vi "valve_controll.vi"() -> ()   [LabVIEW 2011]
uses:
  <vilib>/LabVIEW Interface for Arduino/Type Defs/Pin Mode.ctl
  <vilib>/LabVIEW Interface for Arduino/LabVIEW Interface for Arduino.lvlib
panel:
  in  "Cooling Down Time (min)":dbl=20.0 caption="Time Target (s)"
  out "Elapsed Time (s)":dbl
  out "x > y?":bool
  in  "Back Valve Time (min)":dbl=20.0 caption="Time Target (s)"
  in  "Chromatogram Time (min)":dbl=20.0 caption="Time Target (s)"
  in  "VISA resource":refnum<visa-resource-name>
  in  "Digital I/O Pin":u8
  in  "Value (0)":u8
  in  "Stop":bool
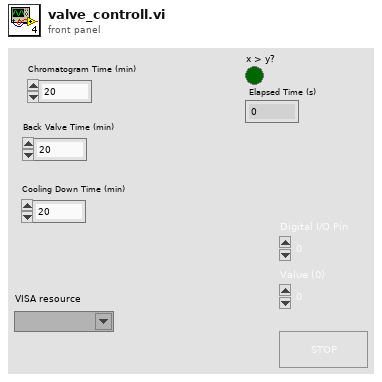
[diagram p1: front panel]
types:
  T1 = typedef "LabVIEW Interface for Arduino.lvlib/Pin Mode.ctl" = enum8{"Input", "Output"}
  T2 = typedef "LabVIEW Interface for Arduino.lvlib/Arduino Resource.ctl" = cluster{"VISA resource":refnum<visa-resource-name>, "Board Type":T3, "Connection Type":enum8{"USB / Serial"}, "Bytes Per Packet (15)":u8}
  T3 = typedef "LabVIEW Interface for Arduino.lvlib/Board Type.ctl" = enum16{"Uno", "Dimuelanove w/Atmega 328", "Mega 2560"}
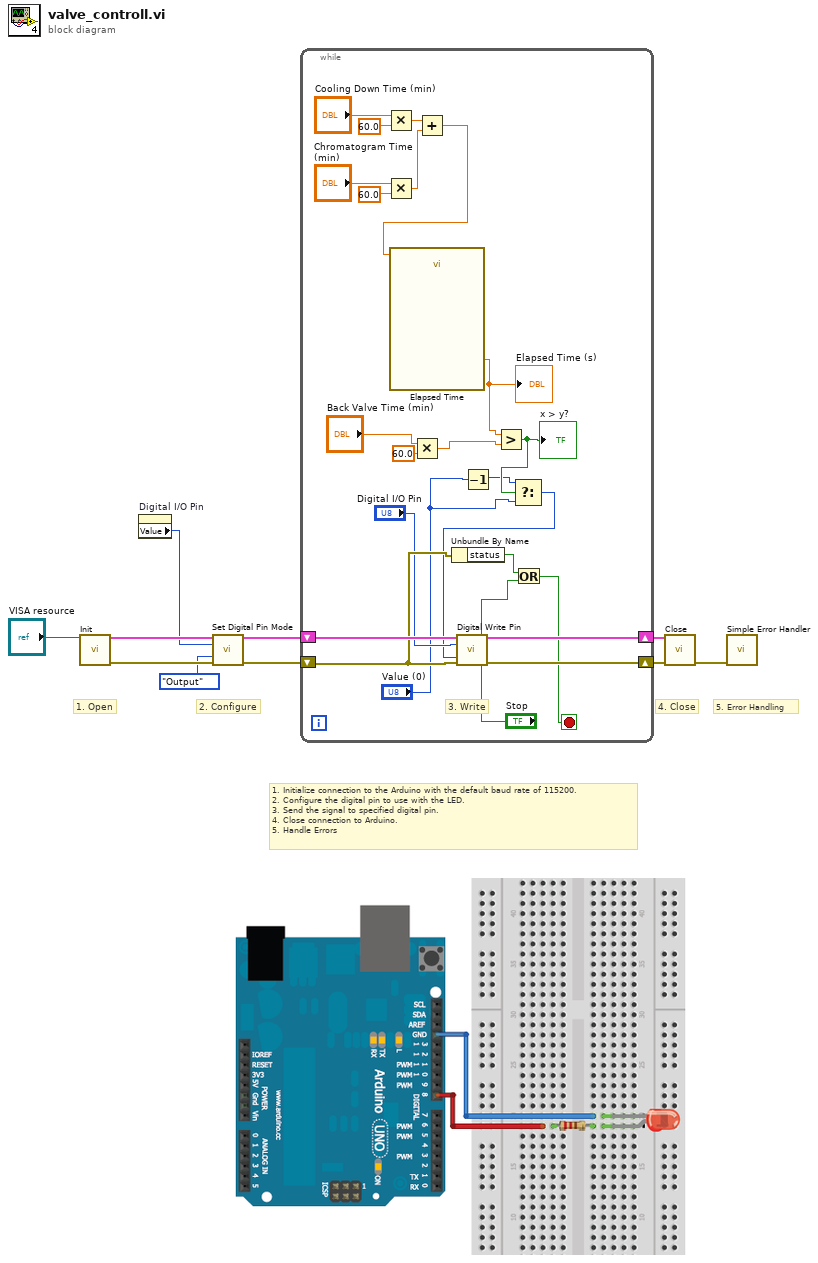
[diagram p0: block diagram]
diagram:
  # "5. Error Handling"
  # "4. Close"
  # "2. Configure"
  # "1. Open"
  # "1. Initialize connection to the Arduino with the default baud rate of 115200.\n2. Configure the digital pin to use with the LED.\n3. Send the signal to specified digital pin.\n4. Close connection to Arduino.\n5. Handle Errors"
  n1 = call <vilib>:"Init.vi"("VISA resource"="VISA resource") -> ("Arduino Resource"=w7:T2, "error out"=w6:errorcluster)  [unwired: 17 in]
  n2 = property on="Digital I/O Pin" class="DigNum (strict)"() -> ("Value"=w1:u8)  [unwired: 2 in, 2 out]
  n3 = call <vilib>:"Set Digital Pin Mode.vi"("Arduino Resource"=w7, "Digital I/O Pin"=w1, "Pin Mode (Input)"=Pin_Mode."Output", "error in"=w6) -> ("Arduino Resource"=w5:T2, "error out"=w4:errorcluster)  [unwired: 10 in]
  n4 = while {
    shift-right: [w33] -> w9
    shift-left: w5 -> [w31]
    shift-right: [w32] -> w8
    shift-left: w4 -> [w29]
    stop <- w27 stop-if-true
    # "3. Write"
    n5 = Multiply(x="Cooling Down Time (min)", y=60.0) -> (x*y=w13:dbl)
    n6 = Multiply(x="Chromatogram Time (min)", y=60.0) -> (x*y=w12:dbl)
    n7 = Multiply(x="Back Valve Time (min)", y=60.0) -> (x*y=w17:dbl)
    n8 = Add(x=w13, y=w12) -> (x+y=w11:dbl)
    n9 = call "Elapsed Time"("Time Target (s)"=w11) -> ("Elapsed Time (s)"=w26:dbl)  [unwired: 11 in, 7 out]
    "Elapsed Time (s)" <- w26
    n10 = Unbundle By Name(w29) -> ("status"=w30:bool)
    n11 = Decrement(x="Value (0)") -> (x-1=w22:u8)
    n12 = Greater?(x=w26, y=w17) -> (0:w25:bool)
    "x > y?" <- w25
    n13 = Select(t=w22, s=w25, f="Value (0)") -> (s? t:f=w23:u8)
    n14 = call <vilib>:"Digital Write Pin.vi"("Arduino Resource"=w31, "Digital I/O Pin (0)"="Digital I/O Pin", "Value (0)"=w23, "error in"=w29) -> ("Arduino Resource"=w33:T2, "error out"=w32:errorcluster)  [unwired: 10 in]
    n15 = Or(x=w30, y="Stop") -> (x .or. y?=w27:bool)
  }
  n16 = call <vilib>:"Close.vi"("Arduino Resource"=w9, "error in"=w8) -> ("error out"=w10:errorcluster)  [unwired: 13 in]
  n17 = call <vilib>:"Simple Error Handler.vi"("error in (no error)"=w10) -> ()  [unwired: 4 in, 5 out]
